vi "Timestamp_Creator.vi"(7 "Timestamp Type":enum16{"Base", "Base +/- Rand(Delta T)"}(ring), 8 "error in (no error)":errorcluster, 9 "Delta T (ns)":u64=1000000, 10 "Base Relative Time (ns)":u64=33000000, 11 "Previous Time (ns)":u64=33000000) -> (0 "error out":errorcluster, 3 "Next Time (ns)":u64=33000000)   [LabVIEW 2020]
uses:
  <vilib>/numeric/Random Number (Range) I64.vi
  <vilib>/numeric/sub_Random U32.vi
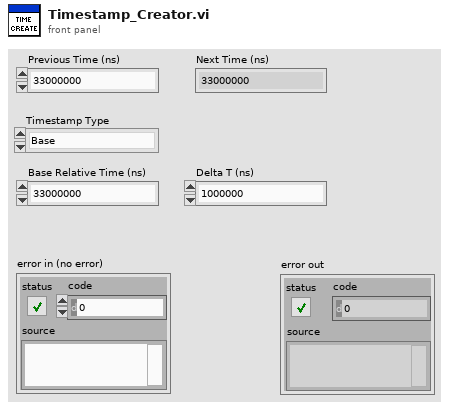
[diagram p1: front panel]
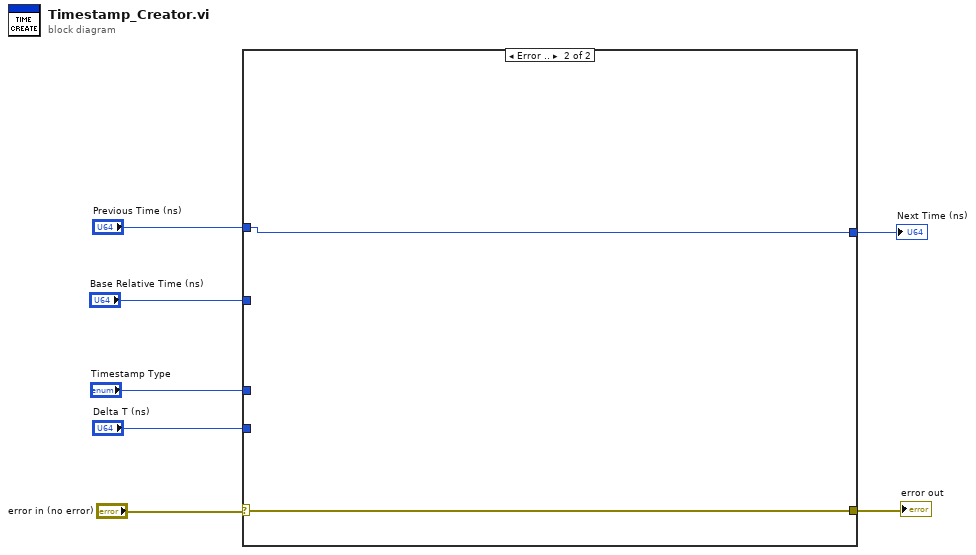
[diagram p0: block diagram]
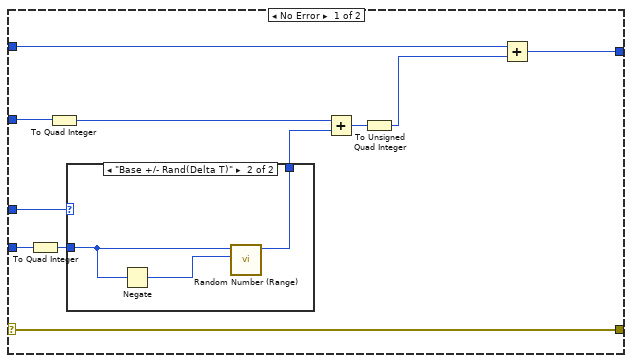
[diagram p2: hidden frame]
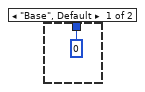
[diagram p3: hidden frame]
diagram:
  n1 = case shown="Error .." "error in (no error)" {
    selector: "error in (no error)" -> [w10 w24]
    tunnel: "Delta T (ns)" -> [w18 _]
    tunnel: "Base Relative Time (ns)" -> [w16 _]
    tunnel: "Previous Time (ns)" -> [w12 w23]
    tunnel: [w10 w24] -> w3
    tunnel: "Timestamp Type" -> [w9 _]
    tunnel: [w8 w23] -> w1
    frame No Error {
      n2 = To Quad Integer(1:w18) -> (0:w17:i64)
      n3 = To Quad Integer(1:w16) -> (0:w15:i64)
      n4 = case shown="\"Base +/- Rand(Delta T)\"" w9 {
        tunnel: w17 -> [_ w22]
        tunnel: [i64 0 ("number") w20] -> w14
        frame "Base", Default {
        }
        frame "Base +/- Rand(Delta T)" {
          n5 = Negate(x=w22) -> (-x=w21:i64)
          n6 = call-poly <vilib>:"Random Number (Range).vi"("lower bound (-100)"=w21, "upper bound (100)"=w22) -> ("number"=w20:i64)  [unwired: 9 in]
        }
      }
      n7 = Add(x=w15, y=w14) -> (x+y=w13:i64)
      n8 = To Unsigned Quad Integer(1:w13) -> (0:w11:u64)
      n9 = Add(x=w12, y=w11) -> (x+y=w8:u64)
    }
    frame Error {
    }
  }
  "error out" <- w3
  "Next Time (ns)" <- w1
